vi "ft_with_2f.vi"() -> ()   [LabVIEW 2021]
uses:
  <vilib>/express/express analysis/Spectral/Block/exnSpectralBlock spectral measurements PSD poly.vi
  <vilib>/express/express analysis/Spectral/Block/exnSpectralBlock spectral measurements PSD DDT.vi
  <vilib>/express/express analysis/Spectral/XNode/ExpressSpectralMeasurementsBlockNode.xnode
panel:
  out "Waveform Graph 2":dynamicdata(graph)
  in  "Mirror speed":dbl
  in  "speed of light":dbl
  in  "time":dbl
  in  "distance to moving arm":dbl
  out "Waveform Graph":dynamicdata(graph)
  in  "Amplitude":dbl=1.0
  in  "distance to arm":dbl
  in  "Wavelength":dbl
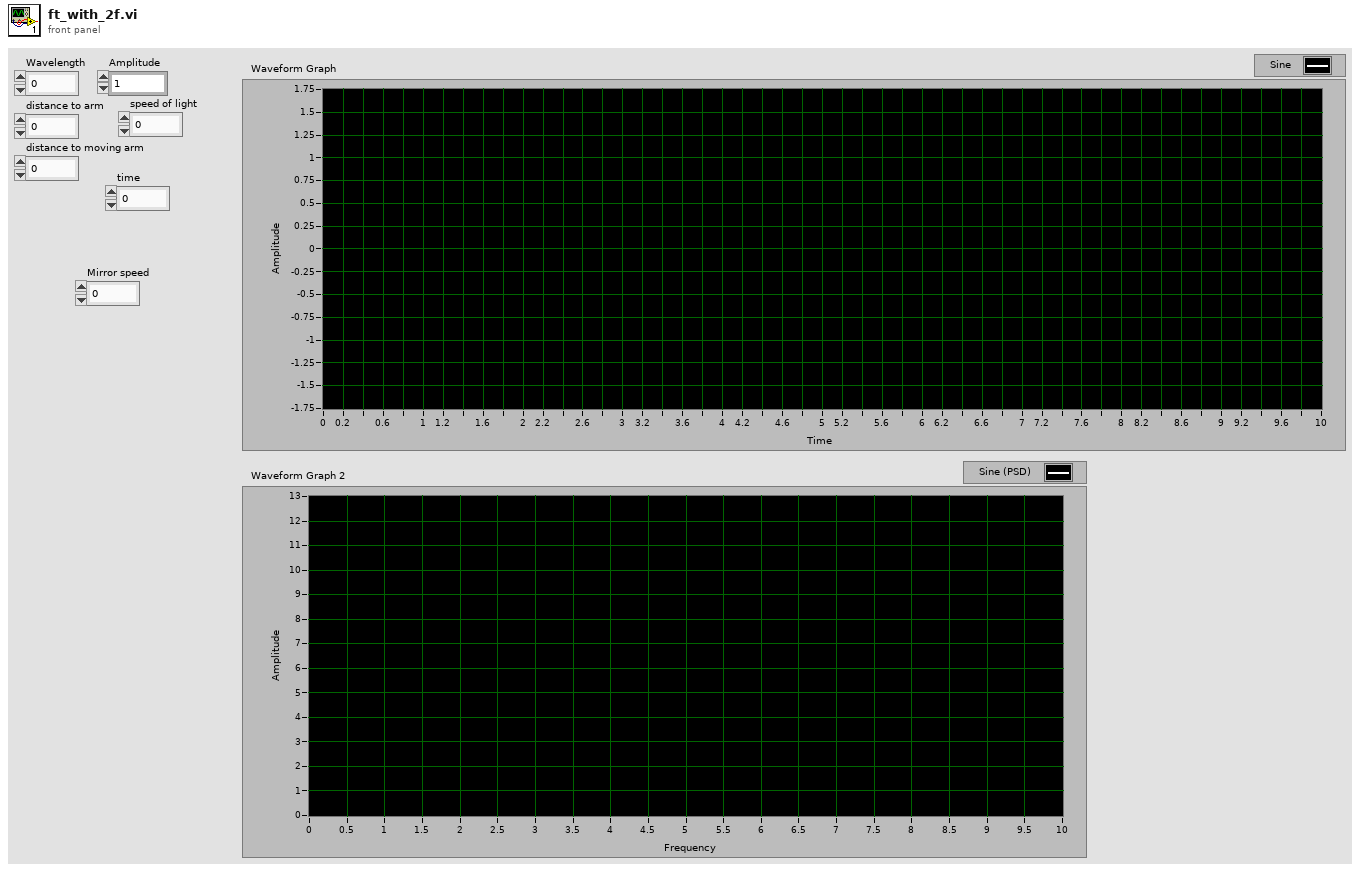
[diagram p1: front panel]
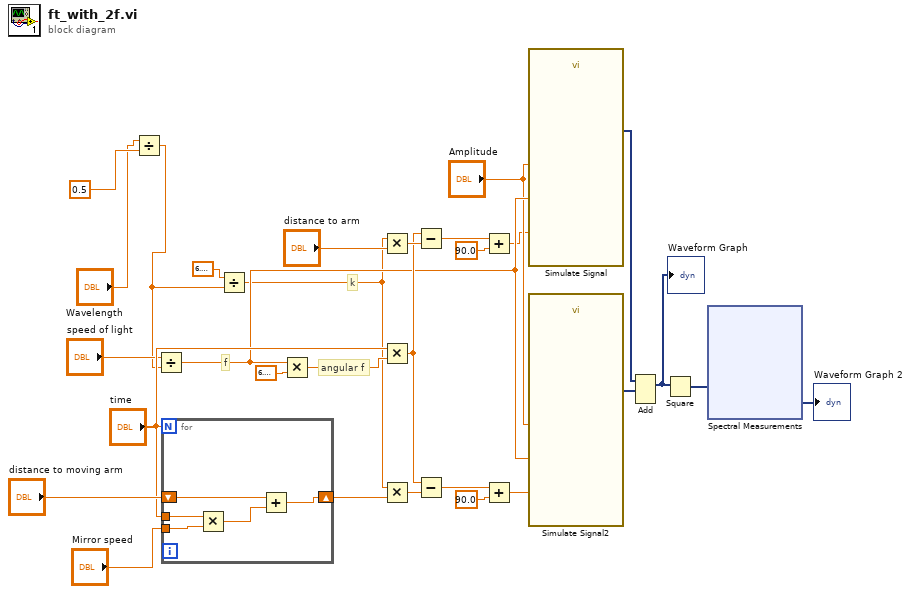
[diagram p0: block diagram]
diagram:
  # "angular f"
  # "f"
  # "k"
  n1 = Divide(x="Wavelength", y=0.5) -> (x/y=w1:dbl)
  n2 = Divide(x="speed of light", y=w1) -> (x/y=w15:dbl)
  n3 = for {
    N: "time" -> [_]
    shift-right: [w33] -> w17
    shift-left: "distance to moving arm" -> [w34]
    tunnel: "time" -> [w32]
    tunnel: "Mirror speed" -> [w31]
    n4 = Multiply(x=w32, y=w31) -> (x*y=w30:dbl)
    n5 = Add(x=w34, y=w30) -> (x+y=w33:dbl)
  }
  n6 = Divide(x=6.283185307179586, y=w1) -> (x/y=w10:dbl)
  n7 = Multiply(x=w15, y=6.283185307179586) -> (x*y=w23:dbl)
  n8 = Multiply(x=w10, y="distance to arm") -> (x*y=w22:dbl)
  n9 = Multiply(x="time", y=w23) -> (x*y=w21:dbl)
  n10 = Multiply(x=w10, y=w17) -> (x*y=w20:dbl)
  n11 = Subtract(x=w21, y=w22) -> (x-y=w9:dbl)
  n12 = Subtract(x=w21, y=w20) -> (x-y=w5:dbl)
  n13 = Add(x=w9, y=90.0) -> (x+y=w8:dbl)
  n14 = Add(x=w5, y=90.0) -> (x+y=w4:dbl)
  n15 = call "Simulate Signal"("Frequency"=w15, "Amplitude"="Amplitude", "Phase"=w8) -> ("Sine"=w29:dynamicdata)  [unwired: 11 in, 1 out]
  n16 = call "Simulate Signal2"("Frequency"=w15, "Amplitude"="Amplitude", "Phase"=w4) -> ("Sine"=w28:dynamicdata)  [unwired: 11 in, 1 out]
  n17 = Add(1:w28, 2:w29) -> (0:w12:dynamicdata)  [unwired: 1 in, 1 out]
  "Waveform Graph" <- w12
  n18 = Square(x=w12) -> (x^2=w11:dynamicdata)
  n19 = xnode "Spectral Measurements"("Signals"=w11) -> ("PSD"=→"Waveform Graph 2":dynamicdata)  [unwired: 1 in, 1 out]
